vi "route_queue.vi"(7 "set":enum16{"reset", "write"}(ring), 11 "route":T1[](array[typedef])) -> (2 "read":T1[](array[typedef]))   [LabVIEW 2019]
uses:
  move_cluster.ctl
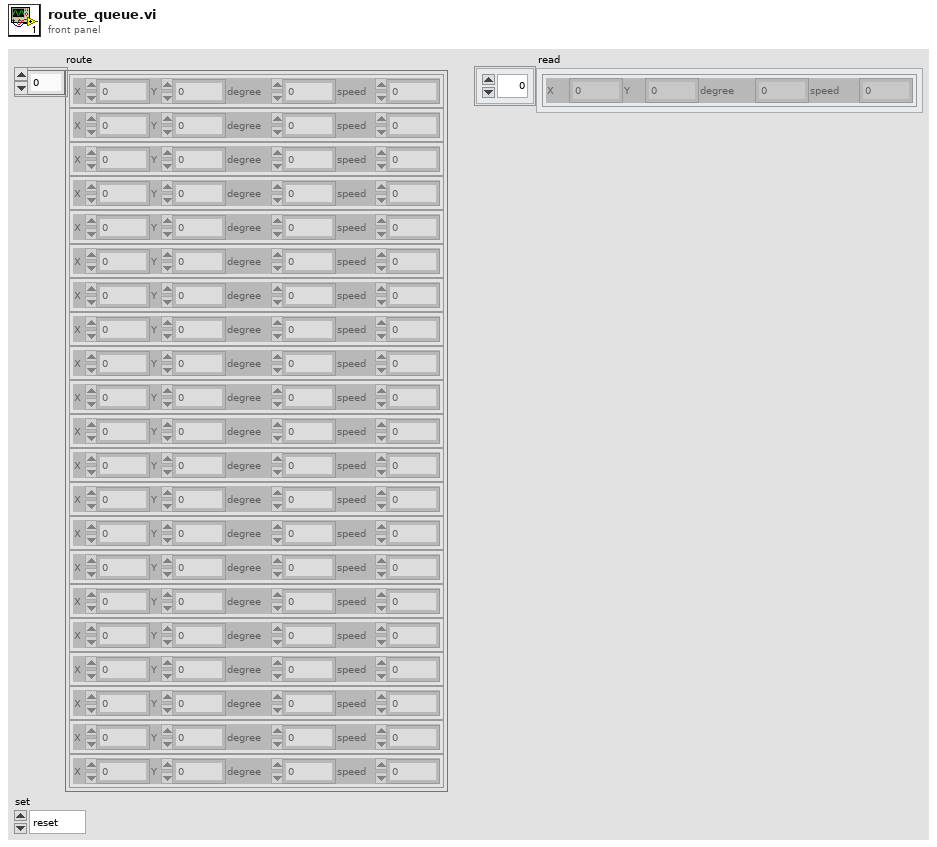
[diagram p1: front panel]
types:
  T1 = typedef "move_cluster.ctl" = cluster{"X":dbl, "Y":dbl, "degree":dbl, "speed":dbl}
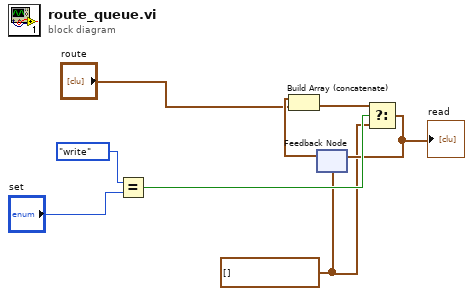
[diagram p0: block diagram]
diagram:
  w1 = T1[] [] ("route")
  n1 = Equal?(x=enum16{"reset", "write"}."write" ("Enum"), y="set") -> (x = y?=w4:bool)
  n2 = feedback #1(w1) -> (w7:T1[])
  n3 = Build Array (concatenate)(w7, "route") -> (w3:T1[])
  n4 = Select(t=w3, s=w4, f=w1) -> (s? t:f=w2:T1[])
  "read" <- w2
  n5 = feedback-in #1(w2) -> ()
